vi "Year2017_Question1.vi"() -> ()   [LabVIEW 2015]
panel:
  in  "stop":bool
  out "Distance":dbl
  in  "y2":dbl
  in  "x2":dbl
  in  "y1":dbl
  in  "x1":dbl
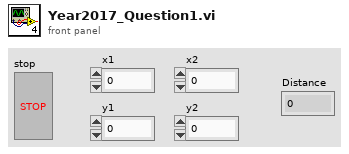
[diagram p1: front panel]
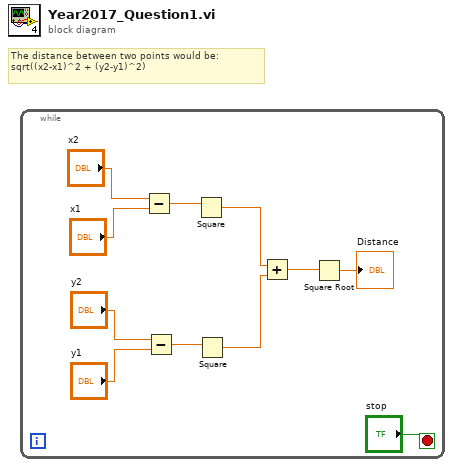
[diagram p0: block diagram]
diagram:
  # "The distance between two points would be:\nsqrt((x2-x1)^2 + (y2-y1)^2)"
  n1 = while {
    stop <- "stop" stop-if-true
    n2 = Subtract(x="x2", y="x1") -> (x-y=w7:dbl)
    n3 = Subtract(x="y2", y="y1") -> (x-y=w6:dbl)
    n4 = Square(x=w7) -> (x^2=w5:dbl)
    n5 = Square(x=w6) -> (x^2=w4:dbl)
    n6 = Add(x=w5, y=w4) -> (x+y=w3:dbl)
    n7 = Square Root(x=w3) -> (sqrt(x)=→"Distance":dbl)
  }
